vi "搜尋檔案.vi"() -> ()   [LabVIEW 2015]
panel:
  in  "pattern":string="*.vi"
  in  "folder path":path=path "C:/Users/jeff.lin.MINAIK/Desktop/程式"
  out "name":string
  in  "檔名關鍵字":string
  out "所有檔名":string[](array[string])
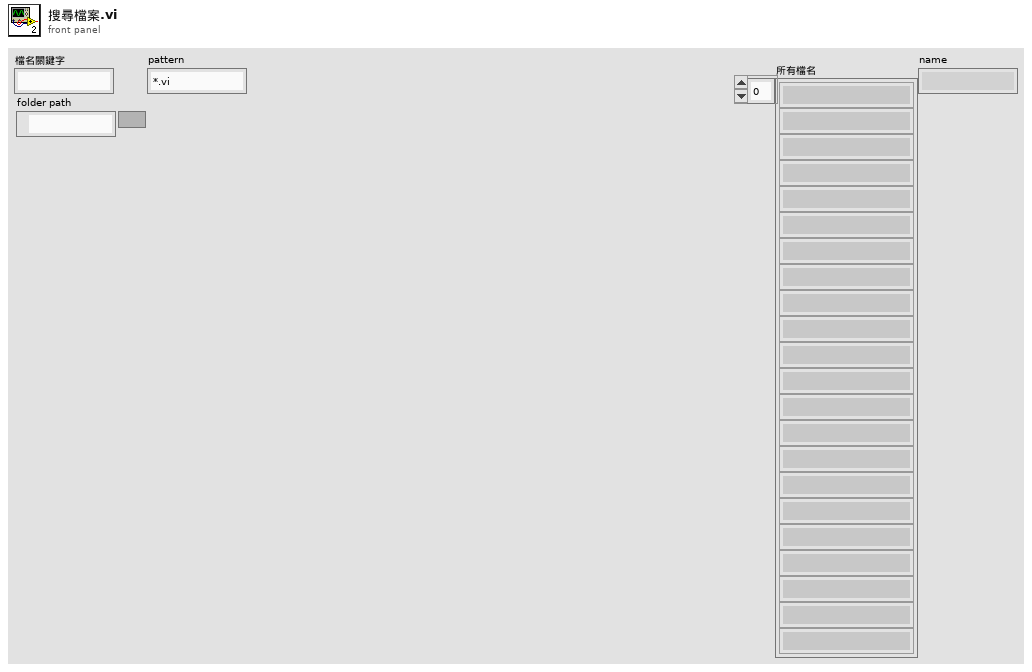
[diagram p1: front panel]
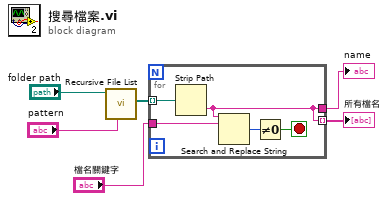
[diagram p0: block diagram]
diagram:
  n1 = call <vilib>:"Recursive File List.vi"("pattern"="pattern", "Folder Path"="folder path") -> ("All Files in Dir"=w5:path[])  [unwired: 5 in, 4 out]
  n2 = for {
    tunnel: w5 -> [w11] mode=indexing
    tunnel: [w7] -> w4 mode=indexing
    tunnel: "檔名關鍵字" -> [w10]
    tunnel: [w7] -> w2
    stop <- w8 stop-if-true
    n3 = Strip Path(path=w11) -> (name=w7:string)  [unwired: 1 out]
    n4 = Search and Replace String(input string=w7, search string=w10) -> (number of replacements=w9:i32)  [unwired: 6 in, 3 out]
    n5 = Not Equal To 0?(x=w9) -> (x != 0?=w8:bool)
  }
  "所有檔名" <- w4
  "name" <- w2
